vi "UCD_Device-Info.vi"(0 "COMPORT":refnum<visa-resource-name>="COM4", 11 "error in (no error)":errorcluster, 12 "OpenSerial(t)":bool, 13 "CloseSerial(t)":bool) -> (2 "Pmic_FwRev":string, 3 "UCD_Device_Info":string, 4 "comport":refnum<visa-resource-name>="COM4", 15 "error out":errorcluster)   [LabVIEW 2018]
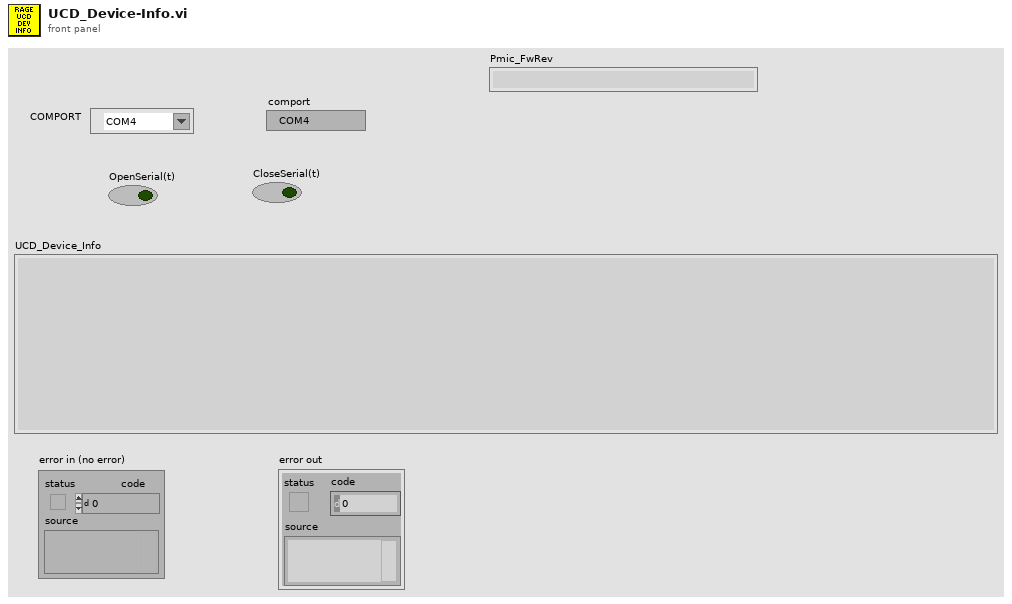
[diagram p1: front panel]
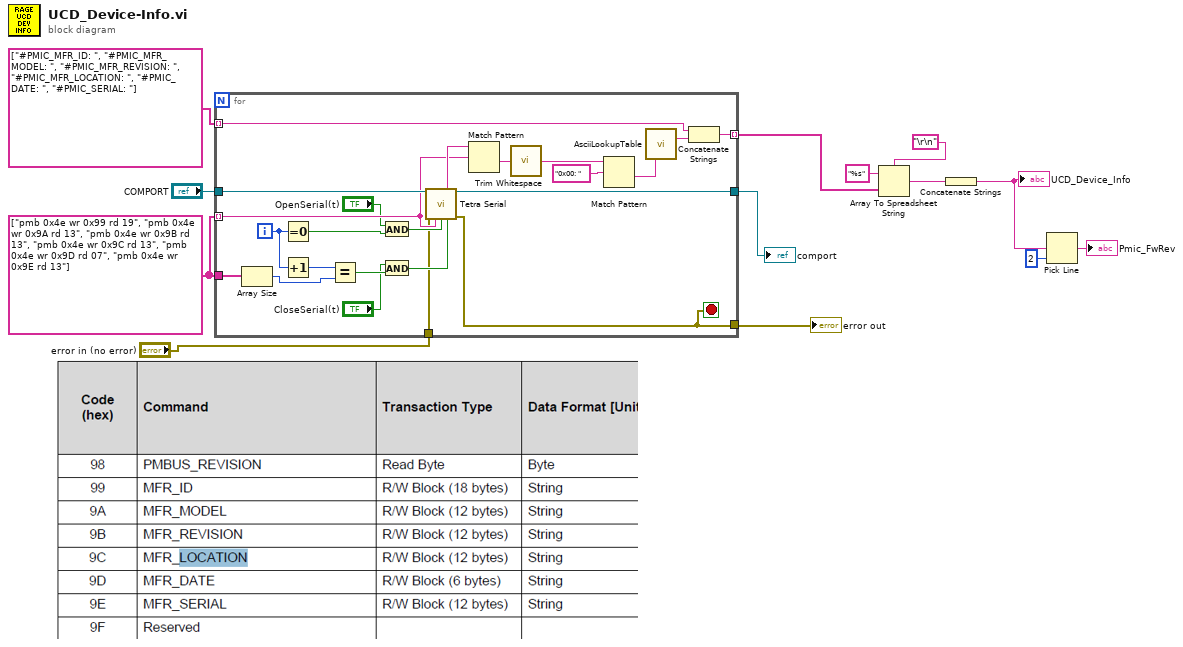
[diagram p0: block diagram]
diagram:
  w12 = string[] ["pmb 0x4e wr 0x99 rd 19", "pmb 0x4e wr 0x9A rd 13", "pmb 0x4e wr 0x9B rd 13", "pmb 0x4e wr 0x9C rd 13", "pmb 0x4e wr 0x9D rd 07", "pmb 0x4e wr 0x9E rd 13"] ("Command ( ; seperation)")
  n1 = for {
    tunnel: "COMPORT" -> [w36]
    tunnel: w12 -> [w29] mode=indexing
    tunnel: w12 -> [w28]
    tunnel: [w21] -> w7 mode=indexing
    tunnel: string[] ["#PMIC_MFR_ID: ", "#PMIC_MFR_MODEL: ", "#PMIC_MFR_REVISION: ", "#PMIC_MFR_LOCATION: ", "#PMIC_DATE: ", "#PMIC_SERIAL: "] ("Command ( ; seperation)") -> [w23] mode=indexing
    tunnel: [w20] -> w10
    tunnel: "error in (no error)" -> [w15]
    tunnel: [w14] -> w8
    i -> [w34]
    stop <- w14 stop-if-true
    n2 = Array Size(array=w28) -> (size(s)=w27:i32)
    n3 = Equal To 0?(x=w34) -> (x = 0?=w35:bool)
    n4 = Increment(x=w34) -> (x+1=w33:i32)
    n5 = Equal?(x=w33, y=w27) -> (x = y?=w32:bool)
    n6 = And(x="OpenSerial(t)", y=w35) -> (x .and. y?=w19:bool)
    n7 = And(x="CloseSerial(t)", y=w32) -> (x .and. y?=w18:bool)
    n8 = call "Tetra Serial.vi"("COMPORT"=w36, "error in (no error)"=w15, "Command"=w29, "Open Ser(t)"=w19, "Close Ser(t)"=w18) -> ("output"=w31:string, "comport"=w20:refnum<visa-resource-name>, "error out"=w14:errorcluster)  [unwired: 6 in, 2 out]
    n9 = Match Pattern(string=w31, regular expression=w29) -> (after substring=w30:string)  [unwired: 1 in, 3 out]
    n10 = call <vilib>:"Trim Whitespace.vi"("string"=w30) -> ("trimmed string"=w26:string)  [unwired: 1 in]
    n11 = Match Pattern(string=w26, regular expression="0x00: ") -> (after substring=w24:string)  [unwired: 1 in, 3 out]
    n12 = call "AsciiLookupTable.vi"("Input 0x ascii"=w24) -> ("result string"=w22:string)  [unwired: 14 in]
    n13 = Concatenate Strings(w23, w22) -> (w21:string)
  }
  "comport" <- w10
  "error out" <- w8
  n14 = Array To Spreadsheet String(delimiter (Tab)="\r\n", array=w7, 3:"%s" ("format string")) -> (spreadsheet string=w5:string)
  n15 = Concatenate Strings(w5) -> (w3:string)
  "UCD_Device_Info" <- w3
  n16 = Pick Line(multi-line string=w3, line index=2) -> (output string=→"Pmic_FwRev":string)  [unwired: 1 in]
